vi "chooseTurnDirection.vi"(6 "KickTarget":dbl[](array[numeric]), 8 "error in (no error)":errorcluster, 9 "Ball":refnum<class "Ball.lvclass">, 10 "Robot":refnum<class "Robot.lvclass">, 11 "KickToSkill in":refnum<class "KickToSkill.lvclass">) -> (0 "error out":errorcluster, 1 "state":T1, 3 "KickToSkill out":refnum<class "KickToSkill.lvclass">)   [LabVIEW 2023, in "KickToSkill.lvclass"]
uses:
  KickToSkill.lvclass
  Robot_class/Robot.lvclass
  C:/Users/ebert/Desktop/roboime/SSL_AI/Object_class/Object.lvclass
  KickToSkill_v3_states.ctl
  Ball_class/Ball.lvclass
  Object_class/Object.lvclass/Object.ctl
  Object_class/Read position(x,y).vi
  <vilib>/Analysis/NI_AALPro.lvlib
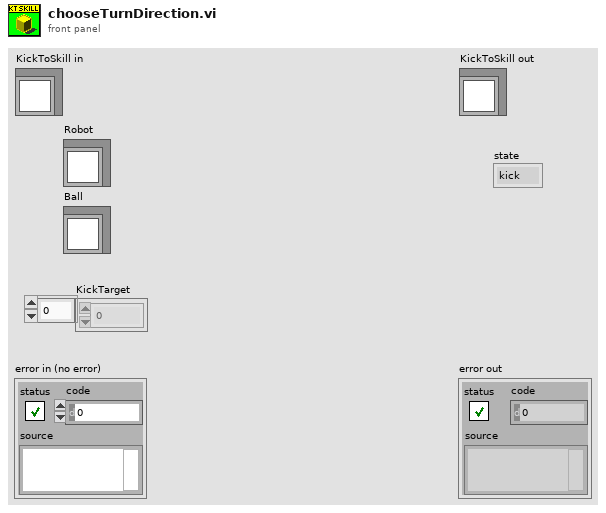
[diagram p1: front panel]
types:
  T1 = typedef "KickToSkill.lvclass/KickToSkill_v3_states.ctl" = enum16{"kick", "align", "turnAntiClockwise", "turnClockwise", "approximate"}
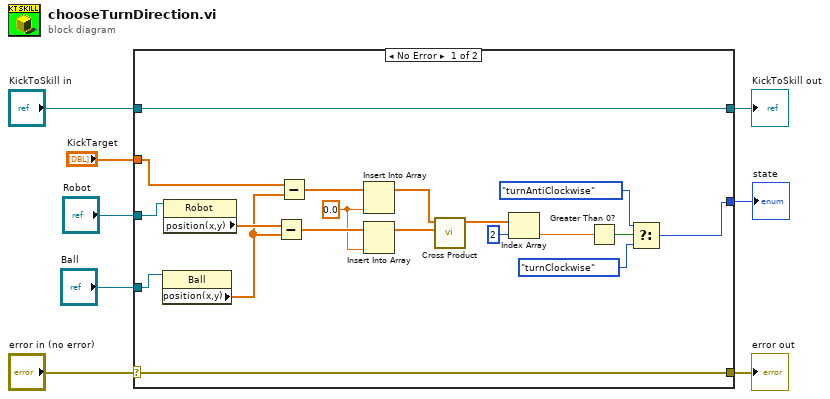
[diagram p0: block diagram]
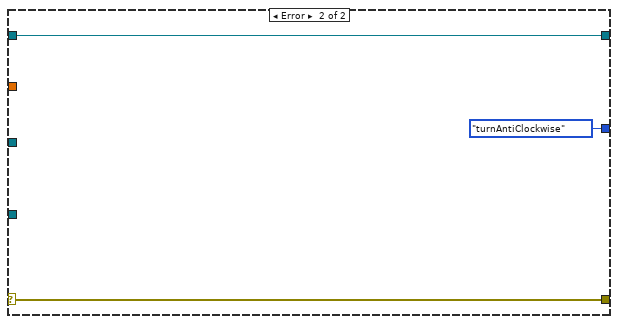
[diagram p2: hidden frame]
diagram:
  n1 = case shown="No Error" "error in (no error)" {
    selector: "error in (no error)" -> [w26 w30]
    tunnel: [w26 w30] -> w7
    tunnel: [w27 w29] -> w5
    tunnel: "KickToSkill in" -> [w27 w29]
    tunnel: "KickTarget" -> [w25 _]
    tunnel: "Robot" -> [w24 _]
    tunnel: "Ball" -> [w23 _]
    tunnel: [w9 KickToSkill_v3_states."turnAntiClockwise" ("state")] -> w1
    frame No Error {
      w18 = 0.0 ("new element/subarray")
      n2 = property class="Ball"(reference=w23) -> ("position(x,y)"=w21:dbl[])  [unwired: 1 in, 2 out]
      n3 = property class="Robot"(reference=w24) -> ("position(x,y)"=w22:dbl[])  [unwired: 1 in, 2 out]
      n4 = Subtract(x=w22, y=w21) -> (x-y=w19:dbl[])
      n5 = Subtract(x=w25, y=w21) -> (x-y=w20:dbl[])
      n6 = Insert Into Array(array=w20, new element=w18) -> (w17:dbl[])  [unwired: 1 in]
      n7 = Insert Into Array(array=w19, new element=w18) -> (w16:dbl[])  [unwired: 1 in]
      n8 = call <vilib>:"Cross Product.vi"("B Vector"=w16, "A Vector"=w17) -> ("Cross Product"=w15:dbl[])  [unwired: 8 in, 1 out]
      n9 = Index Array(array=w15, index=2) -> (element=w13:dbl)
      n10 = Greater Than 0?(x=w13) -> (x > 0?=w12:bool)
      n11 = Select(t=KickToSkill_v3_states."turnAntiClockwise" ("state"), s=w12, f=KickToSkill_v3_states."turnClockwise" ("state")) -> (s? t:f=w9:T1)
    }
    frame Error {
    }
  }
  "error out" <- w7
  "KickToSkill out" <- w5
  "state" <- w1
